vi "Array Elements section.vi"(10 "child strings":string[](array[string]), 11 "indent":i32) -> (3 "Array Elements section":T1)   [LabVIEW 2017, in "DSF Configuration Utility.lvlib"]
uses:
  DSF Configuration Utility.lvlib
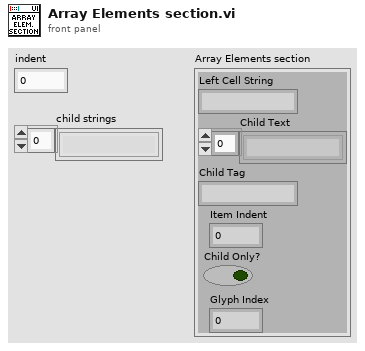
[diagram p1: front panel]
types:
  T1 = cluster{"Left Cell String":string, "Child Text":string[], "Child Tag":string, "Item Indent":i32, "Child Only?":bool, "Glyph Index":i32}
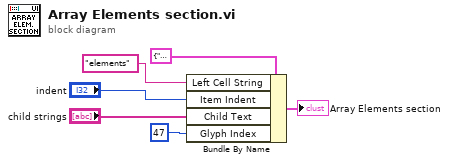
[diagram p0: block diagram]
diagram:
  n1 = Bundle By Name(cluster=T1 {"Left Cell String"="", "Child Text"=[], "Child Tag"="", "Item Indent"=0, "Child Only?"=FALSE, "Glyph Index"=0} ("Item"), "Left Cell String"="elements", "Item Indent"="indent", "Child Text"="child strings", "Glyph Index"=47) -> (→"Array Elements section":T1)
